vi "test Read-Write BIU Configuration.vi"(8 "error in":errorcluster, 11 "TestCase in":refnum<class "Scripting.lvclass">) -> (0 "error out":errorcluster, 3 "TestCase out":refnum<class "Scripting.lvclass">)   [LabVIEW 2020, in "Scripting.lvclass"]
uses:
  Scripting.lvclass
  C:/dev/git/niveristand-custom-device-testing-tools/VeriStandScriptingTestCase/VeriStandScriptingTestCase.lvclass
  Shared/Address.ctl
  Shared/Major Frame Definition.ctl
  Shared/Minor Frame Definition.ctl
  Shared/Message Definition.ctl
  Shared/Message Type.ctl
  Shared/Terminal Endpoint.ctl
  Shared/Parameter Definition.ctl
  Shared/1553 Channel.ctl
  niveristand-custom-device-testing-tools/VeriStandScriptingTestCase/VeriStandScriptingTestCase.lvclass/VeriStandScriptingTestCase.ctl
  niveristand-custom-device-testing-tools/VeriStandScriptingTestCase/Read Target.vi
  NationalInstruments.VeriStand.SystemDefinitionAPI
  <vilib>/addons/_JKI Toolkits/VI Tester/TestCase.llb/TestCase.lvclass
  Scripting/AIM MIL-STD-1553 Scripting.lvlib
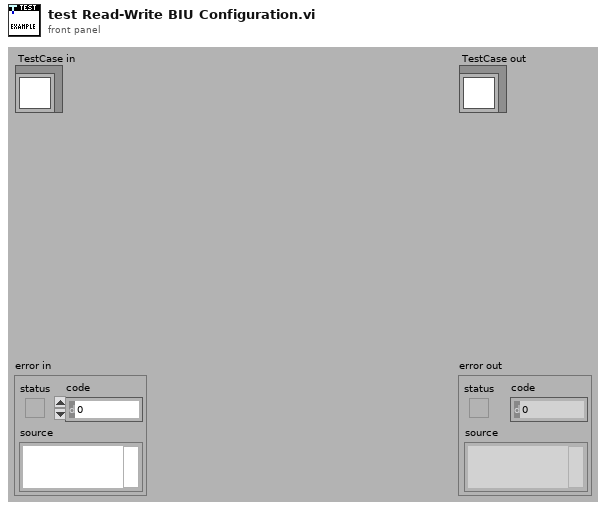
[diagram p1: front panel]
types:
  T1 = typedef "1553 Channel.ctl" = cluster{"HW channel":u16, "terminal addresses":T2[], "terminal names":string[], "acyclic frame names":string[], "major frames":T3[], "minor frames":T4[], "messages":T5[]}
  T2 = typedef "Address.ctl" = u16
  T3 = typedef "Major Frame Definition.ctl" = cluster{"name":string, "minor frames":string[]}
  T4 = typedef "Minor Frame Definition.ctl" = cluster{"name":string, "messages":string[]}
  T5 = typedef "Message Definition.ctl" = cluster{"name":string, "message type":T6, "endpoint Tx":T7, "endpoint Rx":T7, "create timestamp channel":bool, "mode code":u16, "number of words":u16, "parameters":cluster{"name":string, "default value":dbl, "unit":string, "parameter definition":T8}[]}
  T6 = typedef "Message Type.ctl" = string
  T7 = typedef "Terminal Endpoint.ctl" = cluster{"terminal address":T2, "subaddress":T2}
  T8 = typedef "Parameter Definition.ctl" = cluster{"start index":i32, "size (bits)":i32, "encoding":enum16{"BNR", "BCD", "Discrete"}, "signed":bool, "multiplier":dbl, "offset":dbl}
  T9 = typedef "Custom Device API.lvlib/Custom Device Item Ref.ctl" = u64
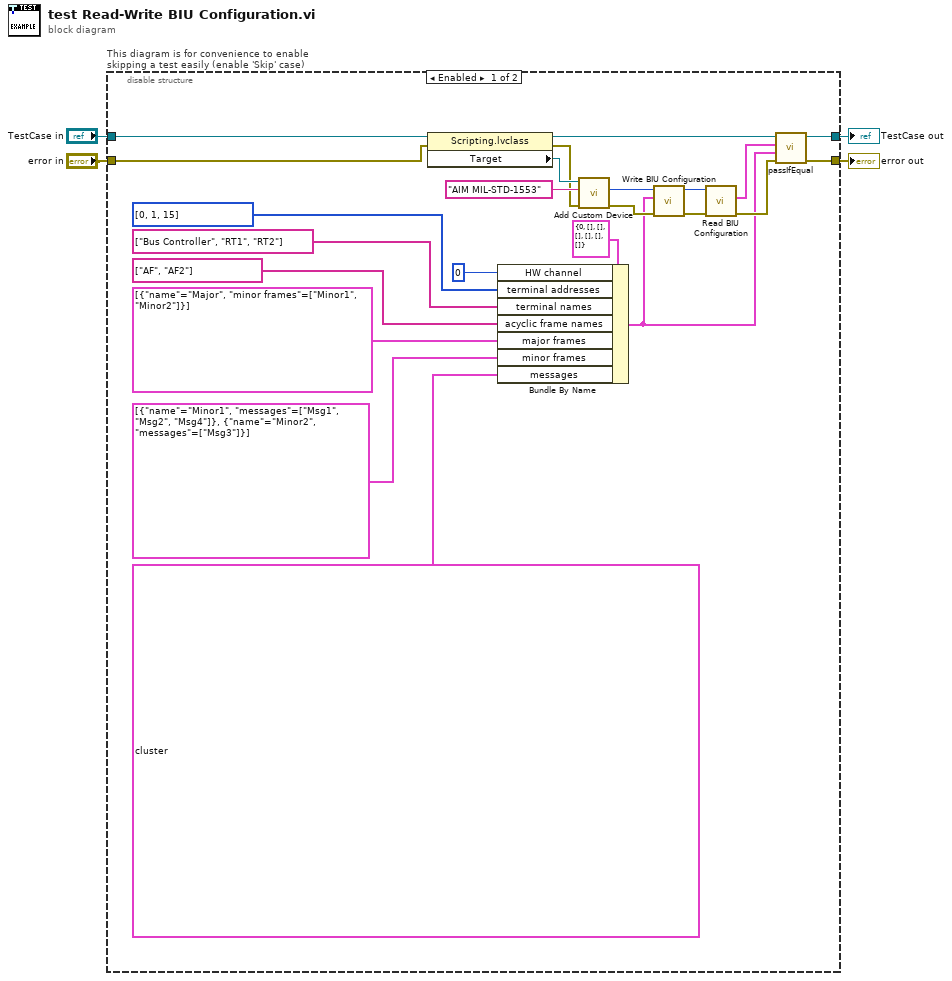
[diagram p0: block diagram]
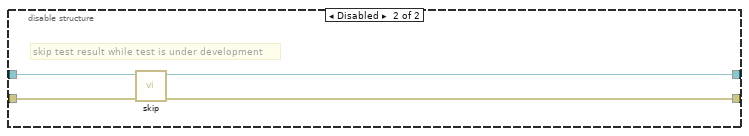
[diagram p2: hidden frame]
diagram:
  n1 = disable-structure "This diagram is for convenience to enable skipping a test easily (enable 'Skip' case)" shown="Enabled" {
    disable-tunnel: "TestCase in" -> [w26 w31]
    disable-tunnel: [w16 w29] -> w1
    disable-tunnel: [w15 w30] -> w3
    disable-tunnel: "error in" -> [w22 w28]
    frame Enabled {
      n2 = property class="Scripting.lvclass"(reference=w26, error in=w22) -> (reference out=w20:refnum<class "Scripting.lvclass">, error out=w21:errorcluster, "Target"=w25:refnum<k24>)
      n3 = Bundle By Name(cluster=T1 {"HW channel"=0, "terminal addresses"=[], "terminal names"=[], "acyclic frame names"=[], "major frames"=[], "minor frames"=[], "messages"=[]}, "HW channel"=u16 0, "terminal addresses"=T2[] [0, 1, 15], "terminal names"=string[] ["Bus Controller", "RT1", "RT2"], "acyclic frame names"=string[] ["AF", "AF2"] ("terminal names"), "major frames"=T3[] [{"name"="Major", "minor frames"=["Minor1", "Minor2"]}], "minor frames"=T4[] [{"name"="Minor1", "messages"=["Msg1", "Msg2", "Msg4"]}, {"name"="Minor2", "messages"=["Msg3"]}], "messages"=T5[] [{"name"="Msg1", "message type"="BC to RT", "endpoint Tx"={"terminal address"=0, "subaddress"=0}, "endpoint Rx"={"terminal address"=0, "subaddress"=0}, "create timestamp channel"=FALSE, "mode code"=0, "number of words"=0, "parameters"=[{"name"="P1", "default value"=1.0, "unit"="", "parameter definition"={"start index"=0, "size (bits)"=16, "encoding"=enum."BNR", "signed"=TRUE, "multiplier"=1.0, "offset"=0.0}}]}, {"name"="Msg2", "message type"="RT to BC", "endpoint Tx"={"terminal address"=0, "subaddress"=0}, "endpoint Rx"={"terminal address"=0, "subaddress"=0}, "create timestamp channel"=TRUE, "mode code"=0, "number of words"=0, "parameters"=[{"name"="P1", "default value"=1.0, "unit"="", "parameter definition"={"start index"=0, "size (bits)"=16, "encoding"=enum."BNR", "signed"=TRUE, "multiplier"=1.0, "offset"=0.0}}]}, {"name"="Msg3", "message type"="RT to RT", "endpoint Tx"={"terminal address"=0, "subaddress"=0}, "endpoint Rx"={"terminal address"=0, "subaddress"=0}, "create timestamp channel"=FALSE, "mode code"=0, "number of words"=0, "parameters"=[]}, {"name"="Msg4", "message type"="MC", "endpoint Tx"={"terminal address"=0, "subaddress"=0}, "endpoint Rx"={"terminal address"=0, "subaddress"=0}, "create timestamp channel"=FALSE, "mode code"=0, "number of words"=0, "parameters"=[]}]) -> (w6:T1)
      n4 = call "Add Custom Device.vi"("error in"=w21, "custom device name"="AIM MIL-STD-1553" ("name"), "target"=w25) -> ("error out"=w23:errorcluster, "custom device ref out"=w24:T9)  [unwired: 6 in, 1 out]
      n5 = call "Write BIU Configuration.vi"("error in"=w23, "biu configuration"=w6, "custom device ref"=w24) -> ("error out"=w18:errorcluster, "custom device ref out"=w19:T9)  [unwired: 7 in]
      n6 = call "Read BIU Configuration.vi"("error in"=w18, "custom device ref"=w19) -> ("error out"=w17:errorcluster, "biu configuration out"=w7:T1)  [unwired: 7 in, 1 out]
      n7 = call-dynamic "passIfEqual.vi"("error in (no error)"=w17, "y"=w6, "x"=w7, "TestCase in"=w20) -> ("error out"=w15:errorcluster, "TestCase out"=w16:refnum<class "Scripting.lvclass">)  [unwired: 6 in]
    }
    frame Disabled {
      # "skip test result while test is under development"
      n8 = call <vilib>:"skip.vi"("error in (no error)"=w28, "TestCase in"=w31) -> ("error out"=w30:errorcluster, "TestCase out"=w29:refnum<class "Scripting.lvclass">)  [unwired: 8 in]
    }
  }
  "error out" <- w3
  "TestCase out" <- w1
